vi "Warm Laser.vi"(8 "error in (no error)":errorcluster, 11 "Laser Process in":refnum<class "Laser Process.lvclass">) -> (0 "error out":errorcluster, 3 "Laser Process out":refnum<class "Laser Process.lvclass">)   [LabVIEW 2022 SP3, in "Laser Process.lvlib" / "Laser Process.lvclass"]
uses:
  Laser Process.lvclass
  Laser Process.lvclass/Laser Process.ctl
  Laser Driver/Laser Driver.lvclass
  XY Stage/Process Actor/Process Framework/Process State Data/Process State Data.lvclass
  Laser State Data/Laser State.ctl
  Laser State Data/Laser State Data.lvclass
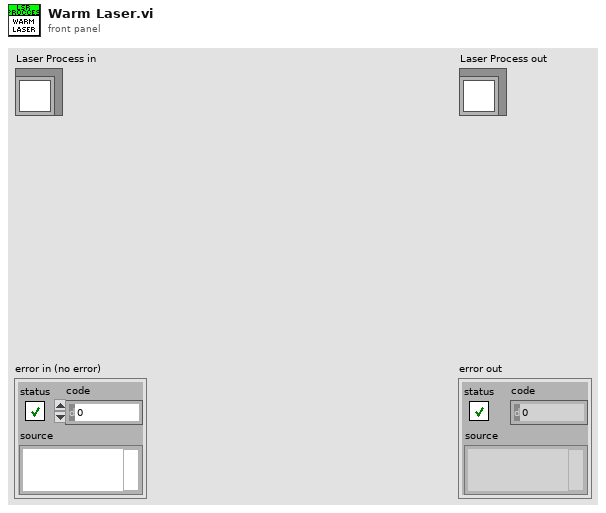
[diagram p1: front panel]
types:
  T1 = typedef "Laser State Data.lvclass/Laser State.ctl" = enum16{"Idle", "Warming", "Ready", "Firing"}
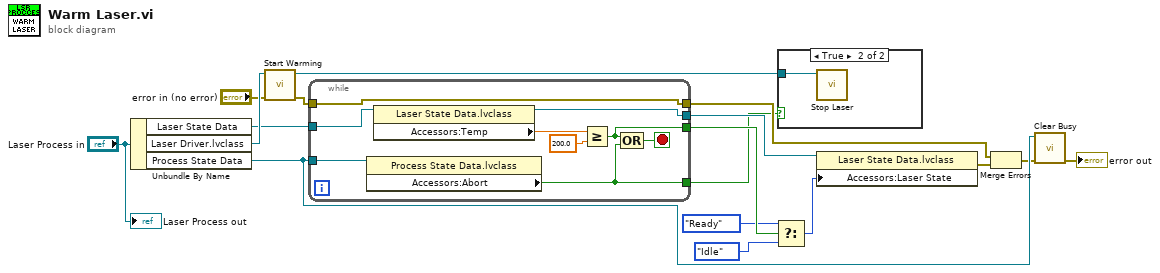
[diagram p0: block diagram]
diagram:
  n1 = Unbundle By Name("Laser Process in") -> ("Laser State Data"=w12:refnum<data-value>, "Laser Driver.lvclass"=w16:refnum<class "Laser Driver.lvclass">, "Process State Data"=w5:refnum<data-value>)
  n2 = call-dynamic "Start Warming.vi"("error in (no error)"="error in (no error)", "Laser Driver in"=w16) -> ("error out"=w13:errorcluster, "Laser Driver out"=w1:refnum<class "Laser Driver.lvclass">)  [unwired: 8 in]
  n3 = while {
    tunnel: w13 -> [w23]
    tunnel: w12 -> [w26]
    tunnel: [w23] -> w11
    tunnel: w5 -> [w22]
    tunnel: [w20] -> w10
    tunnel: [w19] -> w9
    tunnel: [w18] -> w2
    stop <- w21 stop-if-true
    n4 = property class="Process State Data.lvclass"(reference=w22) -> ("Accessors:Abort"=w18:bool)  [unwired: 1 in, 2 out]
    n5 = property class="Laser State Data.lvclass"(reference=w26) -> (reference out=w19:refnum<data-value>, "Accessors:Temp"=w25:dbl)  [unwired: 1 in, 1 out]
    n6 = Greater Or Equal?(x=w25, y=200.0) -> (x >= y?=w20:bool)
    n7 = Compound Arithmetic op=OR(w20, w18) -> (w21:bool)
  }
  n8 = Select(t=Laser_State."Ready" ("Laser State"), s=w10, f=Laser_State."Idle" ("Laser State")) -> (s? t:f=w6:T1)
  n9 = case shown="True" w2 {
    tunnel: w1 -> [_ w27]
    frame False {
    }
    frame True {
      n10 = call-dynamic "Stop Laser.vi"("Laser Driver in"=w27) -> ()  [unwired: 9 in, 2 out]
    }
  }
  n11 = property class="Laser State Data.lvclass"(reference=w9, "Accessors:Laser State"=w6) -> (error out=w3:errorcluster)  [unwired: 1 in, 1 out]
  n12 = Merge Errors(w11, w3) -> (w4:errorcluster)
  n13 = call "Clear Busy.vi"("error in (no error)"=w4, "Process State"=w5) -> ("error out"=→"error out":errorcluster)  [unwired: 8 in, 1 out]
  "Laser Process out" <- "Laser Process in"
